vi "Report_Header.vi"(8 "error in (no error)":errorcluster, 11 "General_Info":T1) -> (0 "error out":errorcluster, 3 "concatenated string":string)   [LabVIEW 2023]
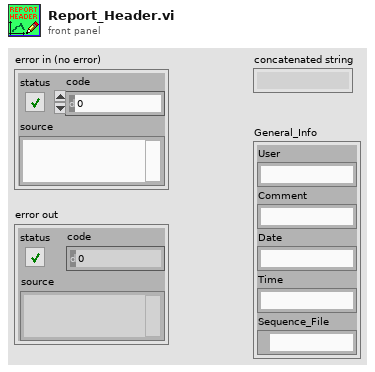
[diagram p1: front panel]
types:
  T1 = cluster{"User":string, "Comment":string, "Date":string, "Time":string, "Sequence_File":path}
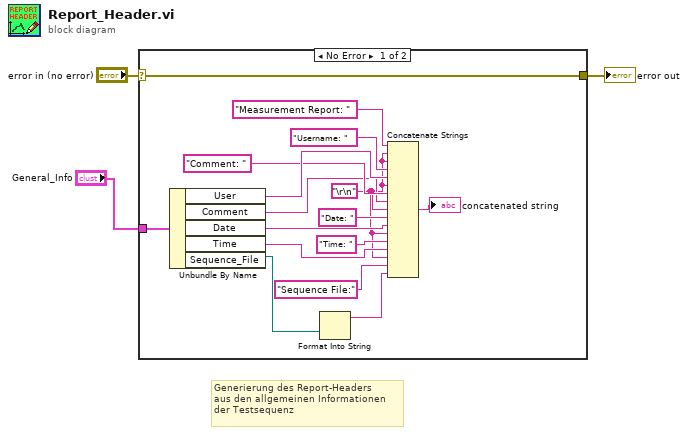
[diagram p0: block diagram]
diagram:
  # "Generierung des Report-Headers\naus den allgemeinen Informationen\nder Testsequenz"
  n1 = case shown="No Error" "error in (no error)" {
    selector: "error in (no error)" -> [w19 w20]
    tunnel: [w19 w20] -> w2
    tunnel: "General_Info" -> [w15 _]
    frame No Error {
      w4 = "\r\n"
      n2 = Unbundle By Name(w15) -> ("User"=w17:string, "Comment"=w13:string, "Date"=w11:string, "Time"=w10:string, "Sequence_File"=w7:path)
      n3 = Format Into String(w7) -> (resulting string=w5:string)  [unwired: 3 in, 1 out]
      n4 = Concatenate Strings("Measurement Report: ", w4, w4, "Username: ", w17, w4, "Comment: ", w13, w4, "Date: ", w11, w4, "Time: ", w10, w4, "Sequence File:" ("string"), w5) -> (→"concatenated string":string)
    }
    frame Error {
    }
  }
  "error out" <- w2
